vi "Get Ref Output.vi"(8 "error in (no error)":errorcluster, 11 "Handle in":i32) -> (0 "error out":errorcluster, 2 "Output":T1, 3 "Handle out":i32)   [LabVIEW 2013, in "Thorlabs_MC2000B.lvlib"]
uses:
  <instrlib>/Thorlabs_MC2000B/Thorlabs_MC2000B.lvlib
  <instrlib>/Thorlabs_MC2000B/Public/Advanced/Output mode.ctl
  Program Files/National Instruments/LabVIEW 2011/instr.lib/Thorlabs_MC2000B/Library/MC2000CommandLibWin64.dll
  <instrlib>/Thorlabs_MC2000B/Library/MC2000CommandLibWin32.dll
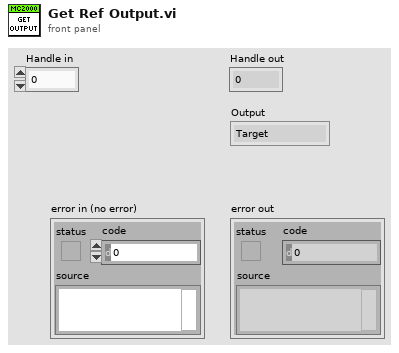
[diagram p1: front panel]
types:
  T1 = typedef "Thorlabs_MC2000B.lvlib/Output mode.ctl" = enum16{"Target", "Actual/Outer", "Inner", "Sum", "Diff"}
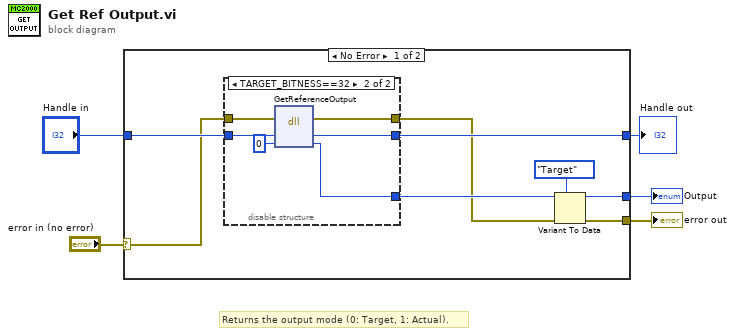
[diagram p0: block diagram]
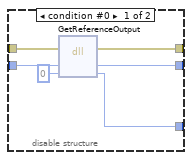
[diagram p2: hidden frame]
diagram:
  # "Returns the output mode (0: Target, 1: Actual)."
  n1 = case shown="No Error" "error in (no error)" {
    selector: "error in (no error)" -> [w6 w27]
    tunnel: [w12 w27] -> w5
    tunnel: [w13 _] -> w3
    tunnel: "Handle in" -> [w10 w26]
    tunnel: [w9 w26] -> w1
    frame No Error {
      n2 = disable-structure shown="TARGET_BITNESS==32" {
        disable-tunnel: w10 -> [w19 w25]
        disable-tunnel: [w18 w24] -> w9
        disable-tunnel: [w17 w23] -> w8
        disable-tunnel: [w16 w22] -> w7
        disable-tunnel: w6 -> [w14 w20]
        frame condition #0 {
          n3 = dll-call lib="D:/Program Files/National Instruments/LabVIEW 2011/instr.lib/Thorlabs_MC2000B/Library/MC2000CommandLibWin64.dll" fn="GetReferenceOutput"(error in=w14, "hdl"=w19, "ref output"=0) -> (error out=w16:errorcluster, "hdl"=w18:i32, "ref output"=w17:i32)  [unwired: 3 in, 1 out]
        }
        frame condition #1 (active) {
          n4 = dll-call lib="C:/Program Files (x86)/National Instruments/LabVIEW 2013/instr.lib/Thorlabs_MC2000B/Library/MC2000CommandLibWin32.dll" fn="GetReferenceOutput"(error in=w20, "hdl"=w25, "ref output"=0) -> (error out=w22:errorcluster, "hdl"=w24:i32, "ref output"=w23:i32)  [unwired: 3 in, 1 out]
        }
      }
      n5 = Variant To Data(error in=w7, type=Output_mode."Target" ("Output"), Variant=w8) -> (data=w13:T1, error out=w12:errorcluster)
    }
    frame Error {
    }
  }
  "error out" <- w5
  "Output" <- w3
  "Handle out" <- w1
